vi "Send CMD_M2.vi"(4 "Travel (mm) M2":dbl, 5 "SERVO ON CMD M2":bool, 6 "Speed (mm/s )M2":dbl, 7 "Mode M2":i32, 9 "Direction M2":bool, 10 "Home Calling M2":bool, 11 "Boolean in":refnum<vi>) -> ()   [LabVIEW 2015]
uses:
  Galobal variable_TI.vi
  Project Setup/Globle Variable/GR_Servo.vi
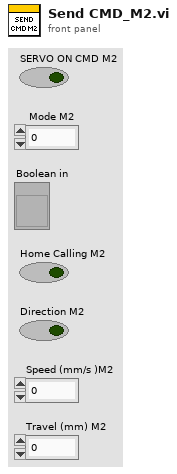
[diagram p1: front panel]
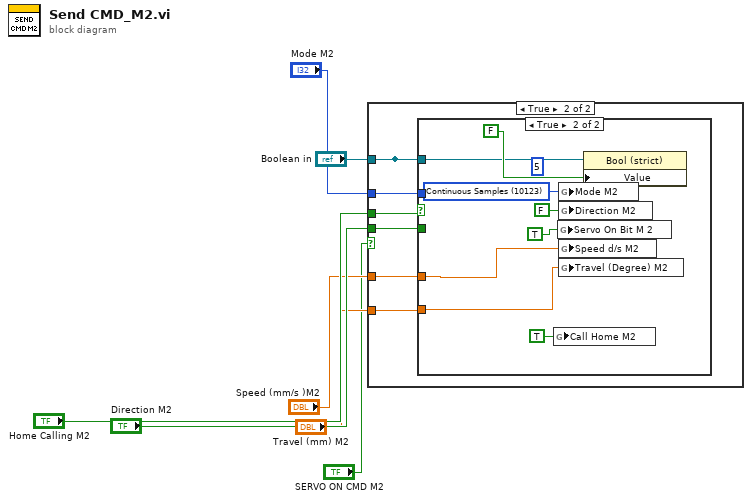
[diagram p0: block diagram]
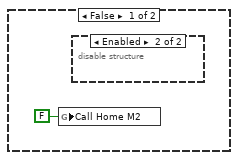
[diagram p2: hidden frame]
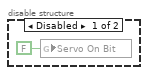
[diagram p3: hidden frame]
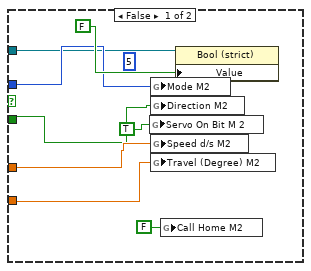
[diagram p4: hidden frame]
diagram:
  n1 = case shown="True" "SERVO ON CMD M2" {
    tunnel: "Speed (mm/s )M2" -> [_ w15]
    tunnel: "Travel (mm) M2" -> [_ w14]
    tunnel: "Direction M2" -> [_ w13]
    tunnel: "Mode M2" -> [_ w12]
    tunnel: "Home Calling M2" -> [_ w11]
    tunnel: "Boolean in" -> [_ w10]
    frame False {
      n2 = global write "Galobal variable_TI.vi" "Call Home M2"(FALSE ("Call Home M1")) -> ()
      n3 = disable-structure shown="Enabled" {
        frame Disabled {
          n4 = global write "GR_Servo.vi" "Servo On Bit"(FALSE ("Servo On Bit")) -> ()
        }
        frame Enabled {
        }
      }
    }
    frame True {
      n5 = case shown="True" w11 {
        tunnel: w15 -> [w21 w29]
        tunnel: w14 -> [w20 w28]
        tunnel: w13 -> [w18 _]
        tunnel: w12 -> [w19 _]
        tunnel: w10 -> [w16 _]
        tunnel: w10 -> [_ w24]
        frame False {
          (unwired) 5 ("index")
          n6 = global write "GR_Servo.vi" "Servo On Bit M 2"(TRUE ("Servo On Bit")) -> ()
          n7 = global write "GR_Servo.vi" "Mode M2"(w19) -> ()
          n8 = global write "GR_Servo.vi" "Direction M2"(w18) -> ()
          n9 = global write "GR_Servo.vi" "Speed d/s M2"(w21) -> ()
          n10 = global write "GR_Servo.vi" "Travel (Degree) M2"(w20) -> ()
          n11 = global write "Galobal variable_TI.vi" "Call Home M2"(FALSE ("Call Home M1")) -> ()
          n12 = property class="Bool (strict)"(reference=w16, "Value"=FALSE ("SERVO ON CMD M2")) -> ()  [unwired: 1 in, 2 out]
        }
        frame True {
          w27 = 10123 items=["Finite Samples"=10178, "Continuous Samples"=10123, "Hardware Timed Single Point"=12522] ("Mode M2")
          (unwired) 5 ("index")
          n13 = global write "Galobal variable_TI.vi" "Call Home M2"(TRUE ("Call Home M1")) -> ()
          n14 = global write "GR_Servo.vi" "Servo On Bit M 2"(TRUE ("Servo On Bit")) -> ()
          n15 = global write "GR_Servo.vi" "Mode M2"(w27) -> ()
          n16 = global write "GR_Servo.vi" "Direction M2"(FALSE ("Direction M2")) -> ()
          n17 = global write "GR_Servo.vi" "Speed d/s M2"(w29) -> ()
          n18 = global write "GR_Servo.vi" "Travel (Degree) M2"(w28) -> ()
          n19 = property class="Bool (strict)"(reference=w24, "Value"=FALSE ("SERVO ON CMD M2")) -> ()  [unwired: 1 in, 2 out]
        }
      }
    }
  }
